vi "I2S Write(David Documentation).vi"(7 "I2S.WL":u16=32 max=32, 8 "I2S.BitCount":u16=31, 9 "Audio Signals":T1, 10 "I2S.PBLRC":bool, 11 "I2S.BCLK IN":bool) -> (3 "I2S.PBDAT OUT":bool)   [LabVIEW 2015]
uses:
  Audio Signals.ctl
panel:
  # "Overview: Write digital audio data."
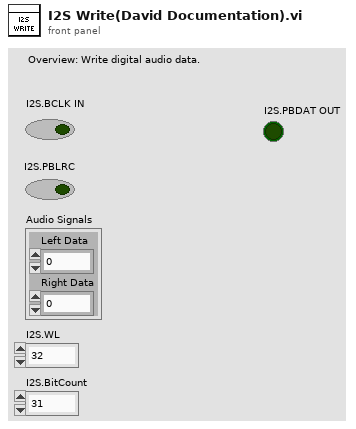
[diagram p1: front panel]
types:
  T1 = typedef "Audio Signals.ctl" = cluster{"Left Data":u32, "Right Data":u32}
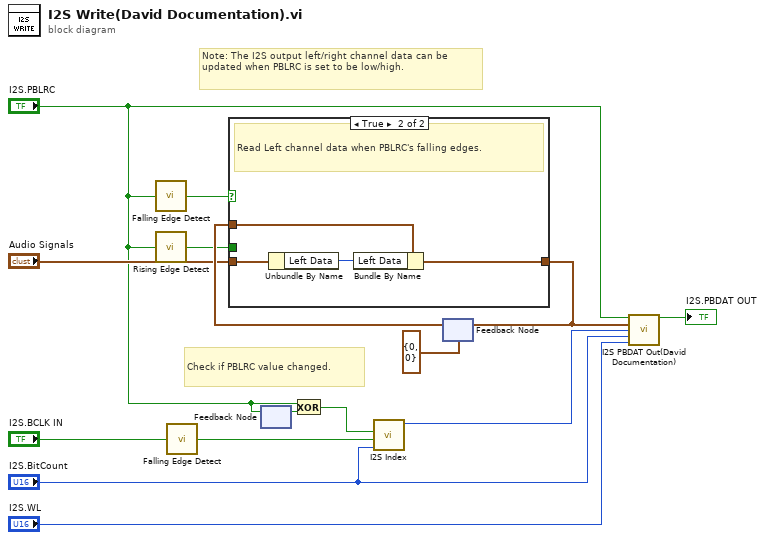
[diagram p0: block diagram]
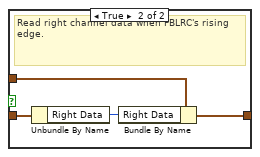
[diagram p3: hidden frame]
diagram:
  # "Check if PBLRC value changed."
  # "Note: The I2S output left/right channel data can be updated when PBLRC is set to be low/high."
  n1 = call "Falling Edge Detect.vi"("Signal"="I2S.PBLRC") -> ("Trigger?"=w6:bool)
  n2 = call "Rising Edge Detect.vi"("Signal"="I2S.PBLRC") -> ("Trigger?"=w1:bool)
  n3 = call "Falling Edge Detect.vi"("Signal"="I2S.BCLK IN") -> ("Trigger?"=w12:bool)
  n4 = feedback #1() -> (w14:bool)  [unwired: 1 in]
  n5 = feedback-in #1("I2S.PBLRC") -> ()
  n6 = Exclusive Or(1:w14, 2:"I2S.PBLRC") -> (0:w13:bool)
  n7 = call "I2S Index.vi"("Bit Count"="I2S.BitCount", "Update"=w12, "Change Channel"=w13) -> ("Value Out"=w10:u16)  [unwired: 8 in]
  n8 = feedback #2(T1 {"Left Data"=0, "Right Data"=0} ("Audio Signals")) -> (w5:T1)
  n9 = case shown="True" w6 {
    tunnel: "Audio Signals" -> [w18 w26]
    tunnel: w5 -> [w19 w28]
    tunnel: [w17 w27] -> w3
    tunnel: w1 -> [w16 _]
    frame False {
      # "No falling edge detected."
      n10 = case shown="False" w16 {
        tunnel: w19 -> [w20 w24]
        tunnel: w18 -> [_ w23]
        tunnel: [w20 w22] -> w17
        frame False {
          # "No rising edge detected."
        }
        frame True {
          # "Read right channel data when PBLRC's rising edge."
          n11 = Unbundle By Name(w23) -> ("Right Data"=w21:u32)
          n12 = Bundle By Name(cluster=w24, "Right Data"=w21) -> (w22:T1)
        }
      }
    }
    frame True {
      # "Read Left channel data when PBLRC's falling edges."
      n13 = Unbundle By Name(w26) -> ("Left Data"=w25:u32)
      n14 = Bundle By Name(cluster=w28, "Left Data"=w25) -> (w27:T1)
    }
  }
  n15 = feedback-in #2(w3) -> ()
  n16 = call "I2S PBDAT Out(David Documentation).vi"("I2S.PBLRC IN"="I2S.PBLRC", "I2S.Data"=w3, "Data Index"=w10, "Bit Count"="I2S.BitCount", "Word Length"="I2S.WL") -> ("I2S.PBDAT OUT"=→"I2S.PBDAT OUT":bool)  [unwired: 10 in]
